vi "elevator.vi"() -> ()   [LabVIEW 2014]
panel:
  out "Direction / -1,0,1":dbl
  out "Initial floor":dbl
  out "Target":dbl
  in  "User input":bool[](array[boolean])
  out "floor limit switch":bool
  out "Floor indicator":bool[](array[boolean])
  in  "Switch button":bool[](array[boolean])
  in  "stop":bool
  out "MOTOR":bool
  # "1"
  # "2"
  # "3"
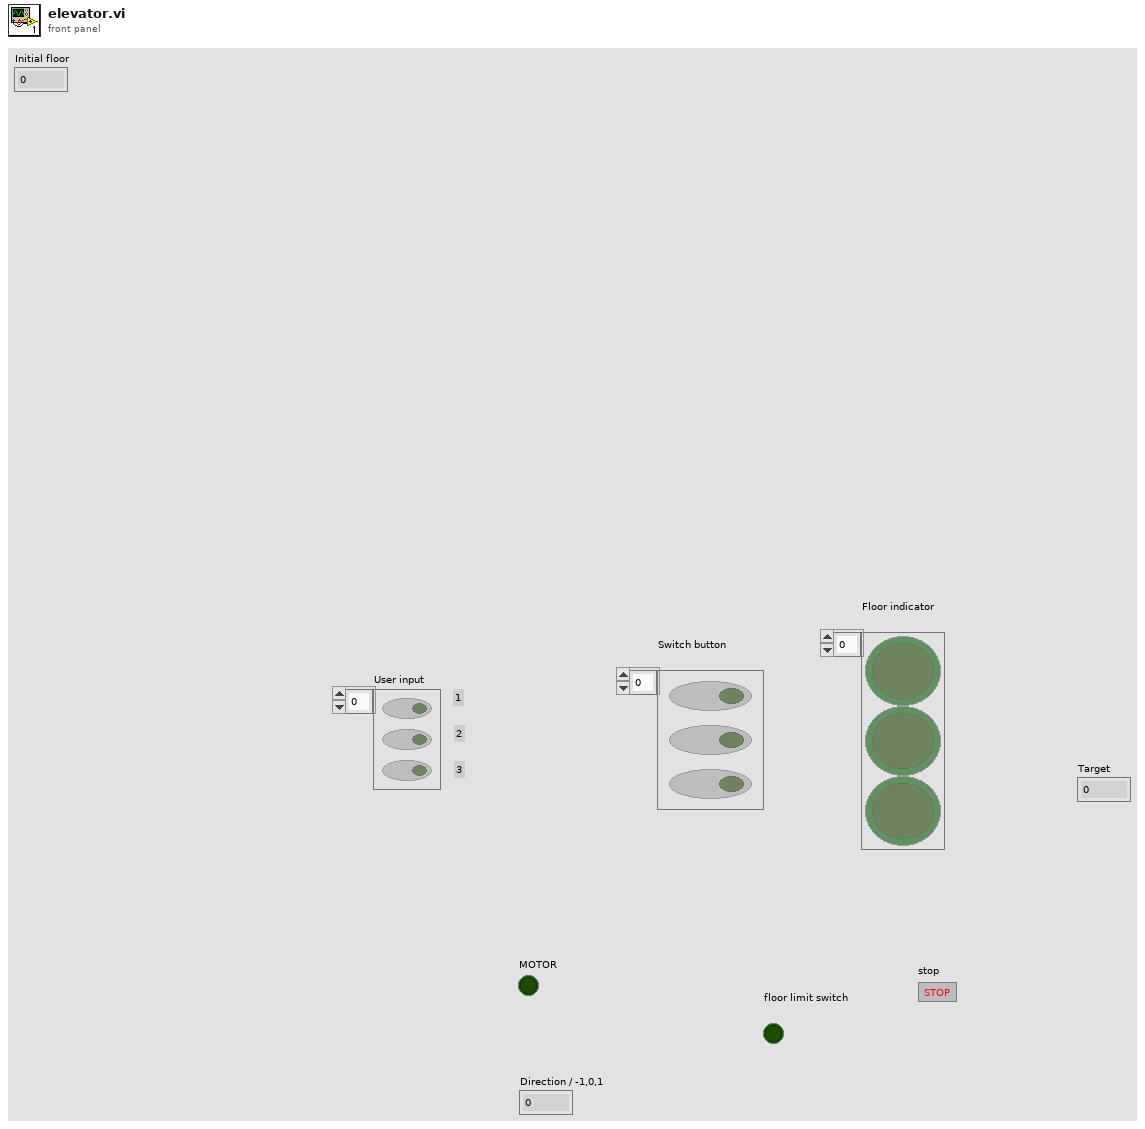
[diagram p1: front panel]
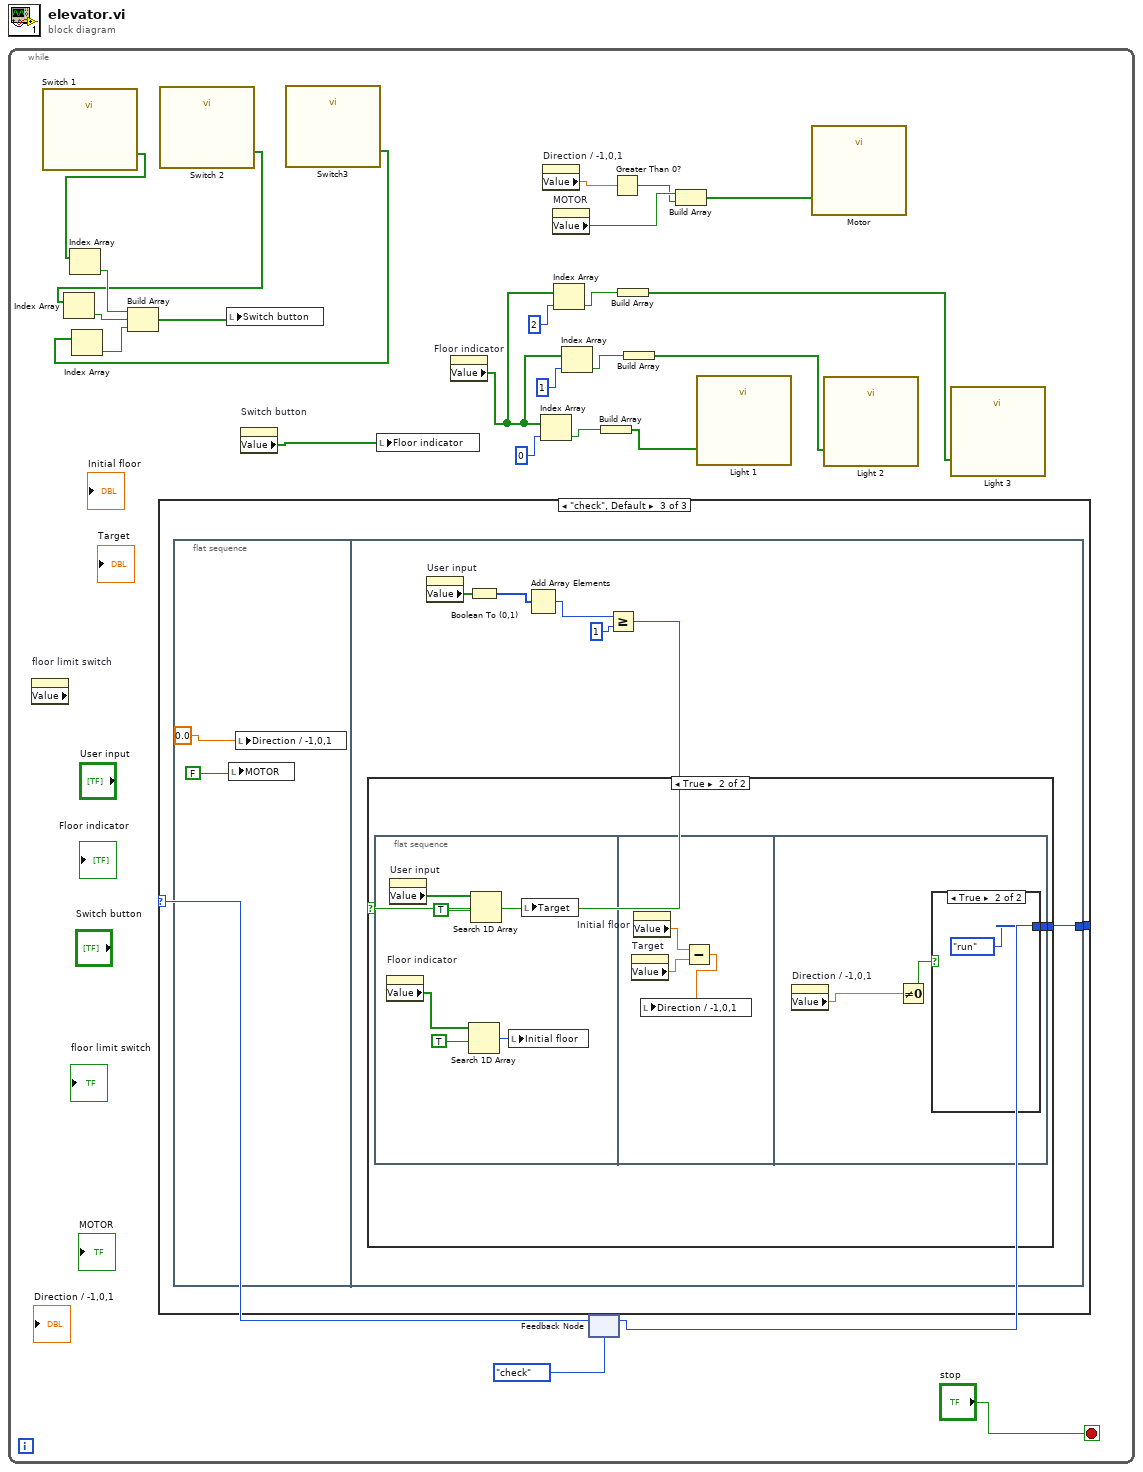
[diagram p0: block diagram]
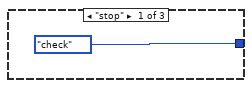
[diagram p2: hidden frame]
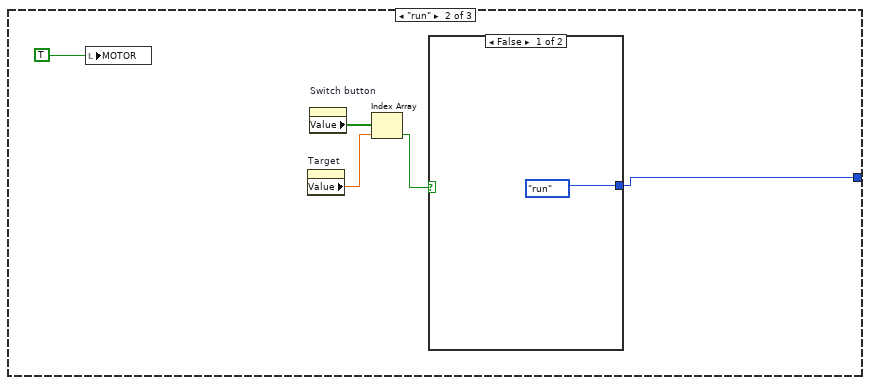
[diagram p3: hidden frame]
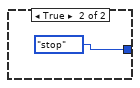
[diagram p4: hidden frame]
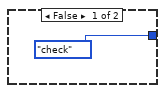
[diagram p5: hidden frame]
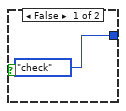
[diagram p6: hidden frame]
diagram:
  n1 = while {
    stop <- "stop" stop-if-true
    n2 = property on="floor limit switch" class="Bool (strict)" props=["Value"]() -> ()  [unwired: 2 in, 3 out]
    n3 = call "Switch 1"() -> ("data"=w9:bool[])  [unwired: 17 in, 2 out]
    n4 = Index Array(array=w9) -> (element=w11:bool)  [unwired: 1 in]
    n5 = call "Switch 2"() -> ("data"=w8:bool[])  [unwired: 17 in, 2 out]
    n6 = Index Array(array=w8) -> (element=w7:bool)  [unwired: 1 in]
    n7 = property on="Switch button" class="Arr (strict)"() -> ("Value"=w22:bool[])  [unwired: 2 in, 2 out]
    n8 = call "Switch3"() -> ("data"=w6:bool[])  [unwired: 17 in, 2 out]
    n9 = Index Array(array=w6) -> (element=w5:bool)  [unwired: 1 in]
    n10 = Build Array(w11, w7, w5) -> (w10:bool[])
    n11 = local write "Switch button"(w10) -> ()
    n12 = local write "Floor indicator"(w22) -> ()
    n13 = property on="Floor indicator" class="Arr (strict)"() -> ("Value"=w16:bool[])  [unwired: 2 in, 2 out]
    n14 = Index Array(array=w16, index=0) -> (element=w20:bool)
    n15 = property on="Direction / -1,0,1" class="DigNum (strict)"() -> ("Value"=w4:dbl)  [unwired: 2 in, 2 out]
    n16 = property on="MOTOR" class="Bool (strict)"() -> ("Value"=w2:bool)  [unwired: 2 in, 2 out]
    n17 = Index Array(array=w16, index=2) -> (element=w14:bool)
    n18 = Index Array(array=w16, index=1) -> (element=w15:bool)
    n19 = feedback #1(enum16{"stop", "run", "check"}."check") -> (w25:enum16{"stop", "run", "check"})
    n20 = case shown="\"check\", Default" w25 {
      tunnel: [enum16{"stop", "run", "check"}."check" w28 w35] -> w23
      frame "stop" {
      }
      frame "run" {
        n21 = local write "MOTOR"(TRUE) -> ()
        n22 = property on="Target" class="DigNum (strict)"() -> ("Value"=w30:dbl)  [unwired: 2 in, 2 out]
        n23 = property on="Switch button" class="Arr (strict)"() -> ("Value"=w31:bool[])  [unwired: 2 in, 2 out]
        n24 = Index Array(array=w31, index=w30) -> (element=w29:bool)
        n25 = case shown="False" w29 {
          tunnel: [enum16{"stop", "run", "check"}."run" enum16{"stop", "run", "check"}."stop"] -> w28
          frame False {
          }
          frame True {
          }
        }
      }
      frame "check", Default {
        n26 = flat-sequence {
          tunnel: [w43] -> w35
          frame #0 {
            n27 = local write "MOTOR"(FALSE) -> ()
            n28 = local write "Direction / -1,0,1"(0.0) -> ()
          }
          frame #1 {
            n29 = property on="User input" class="Arr (strict)"() -> ("Value"=w39:bool[])  [unwired: 2 in, 2 out]
            n30 = Boolean To (0,1)(Boolean=w39) -> (0, 1=w40:i16[])
            n31 = Add Array Elements(numeric array=w40) -> (sum=w42:i16)
            n32 = Greater Or Equal?(x=w42, y=1) -> (x >= y?=w38:bool)
            n33 = case shown="True" w38 {
              tunnel: [enum16{"stop", "run", "check"}."check" w45] -> w43
              frame False {
              }
              frame True {
                n34 = flat-sequence {
                  tunnel: [w57] -> w45
                  frame #0 {
                    n35 = property on="Floor indicator" class="Arr (strict)"() -> ("Value"=w46:bool[])  [unwired: 2 in, 2 out]
                    n36 = property on="User input" class="Arr (strict)"() -> ("Value"=w51:bool[])  [unwired: 2 in, 2 out]
                    n37 = Search 1D Array(1D array=w46, element=TRUE) -> (index of element=w48:i32)  [unwired: 1 in]
                    n38 = Search 1D Array(1D array=w51, element=TRUE) -> (index of element=w49:i32)  [unwired: 1 in]
                    n39 = local write "Initial floor"(w48) -> ()
                    n40 = local write "Target"(w49) -> ()
                  }
                  frame #1 {
                    n41 = property on="Target" class="DigNum (strict)"() -> ("Value"=w53:dbl)  [unwired: 2 in, 2 out]
                    n42 = property on="Initial floor" class="DigNum (strict)"() -> ("Value"=w52:dbl)  [unwired: 2 in, 2 out]
                    n43 = Subtract(x=w52, y=w53) -> (x-y=w54:dbl)
                    n44 = local write "Direction / -1,0,1"(w54) -> ()
                  }
                  frame #2 {
                    n45 = property on="Direction / -1,0,1" class="DigNum (strict)"() -> ("Value"=w56:dbl)  [unwired: 2 in, 2 out]
                    n46 = Not Equal To 0?(x=w56) -> (x != 0?=w55:bool)
                    n47 = case shown="True" w55 {
                      tunnel: [enum16{"stop", "run", "check"}."check" enum16{"stop", "run", "check"}."run"] -> w57
                      frame False {
                      }
                      frame True {
                      }
                    }
                  }
                }
              }
            }
          }
        }
      }
    }
    n48 = feedback-in #1(w23) -> ()
    n49 = Build Array(w20) -> (w19:bool[])
    n50 = Greater Than 0?(x=w4) -> (x > 0?=w1:bool)
    n51 = Build Array(w14) -> (w12:bool[])
    n52 = Build Array(w15) -> (w13:bool[])
    n53 = Build Array(w2, w1) -> (w3:bool[])
    n54 = call "Light 1"("data"=w19) -> ()  [unwired: 17 in, 2 out]
    n55 = call "Motor"("data"=w3) -> ()  [unwired: 17 in, 2 out]
    n56 = call "Light 2"("data"=w13) -> ()  [unwired: 17 in, 2 out]
    n57 = call "Light 3"("data"=w12) -> ()  [unwired: 17 in, 2 out]
  }
